vi "Estimate State-Space Model from FRFs.vi"() -> ()   [LabVIEW 2022 SP3]
doc: "This example demonstrates how to use frequency-domain data to estimate a state-space model. \n\n<B>Instructions:</B>\n1) Run this VI.\n2) Observe how the simulated frequency response matches the measured frequency response.\n3) Change the orders of the models, and observe how these changes affect the estimation error."
uses:
  <vilib>/addons/System Identification/Frequency Domain Estimation.llb/SI Estimate Discrete State-Space Model from FRF (SISO Arbitrary).vi
  <vilib>/addons/System Identification/NI_SysID.lvlib
panel:
  in  "name or relative path":path=path "C:/Users/LAV-UFSC/OneDrive - UFSC/Documents/LAV - TCC/Dados-Experimentos/25-04/frf_2.txt"
  in  "noise subspace (%)":dbl=77.0
  in  "FRF format":T1
  out "Phase Response":cluster{"frequency":dbl[], "amplitude":dbl[]}[](graph)
  out "Magnitude Response":cluster{"frequency":dbl[], "amplitude":dbl[]}[](graph)
  in  "Order":i32=67
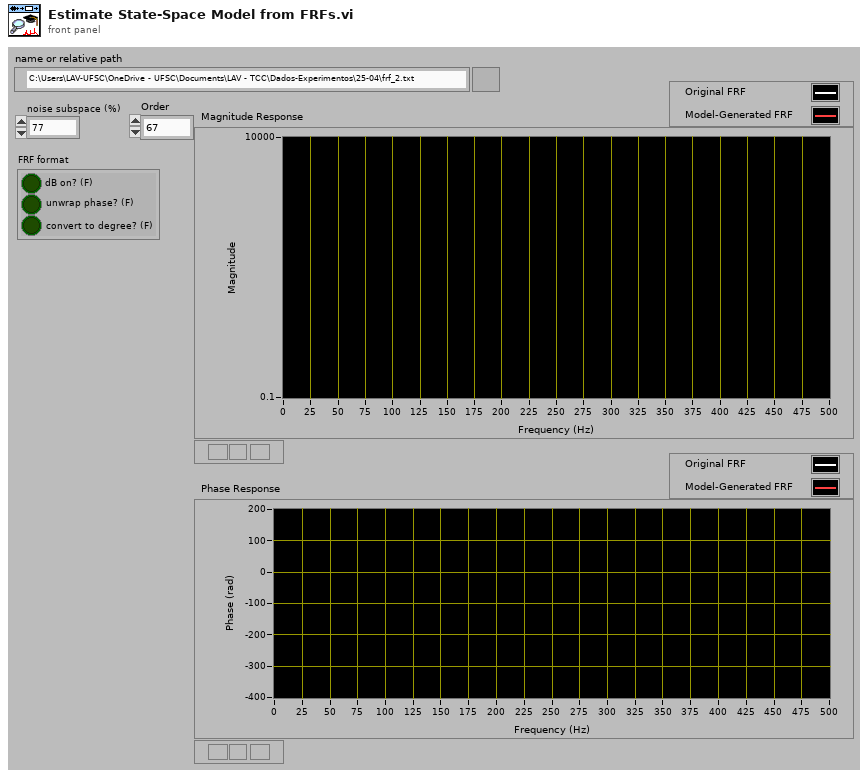
[diagram p1: front panel]
types:
  T1 = cluster{"dB on? (F)":bool, "unwrap phase? (F)":bool, "convert to degree? (F)":bool}
  T2 = cluster{"start frequency":dbl, "end frequency":dbl, "num of freq bins":i32, "interval type":u16}
  T3 = typedef "NI_SysID.lvlib/si_generic model.ctl" = cluster{"attributes":cluster{"version":string, "model type":T4, "input names":string[], "output names":string[], "notes":string}, "coefficients":cluster{"A ":dbl[][][], "B":dbl[][][], "F":dbl[][][], "C":dbl[][][], "D":dbl[][][]}, "std deviations":cluster{"A ":dbl[][][], "B":dbl[][][], "F":dbl[][][], "C":dbl[][][], "D":dbl[][][]}, "coefficients covariance":dbl[][][], "noise variance":dbl[][], "fs":dbl, "system info":cluster{"number of inputs":i32, "number of outputs":i32, "A order":i32[][], "B order":i32[][], "F order":i32[][], "C order":i32[][], "D order":i32[][], "Delays":i32[][]}, "kalman gain":dbl[][], "initial state":dbl[], "trans func":cluster{"betas":dbl[], "alphas":dbl[]}[][], "zeros-poles":cluster{"zeros":cdb[], "poles":cdb[], "gain":dbl}[][], "std of trans func":cluster{"betas":dbl[], "alphas":dbl[]}[][], "std of zeros-poles":cluster{"zeros":cdb[], "poles":cdb[], "gain":dbl}[][], "trans func (noise)":cluster{"betas":dbl[], "alphas":dbl[]}[][], "std of trans func (noise)":cluster{"betas":dbl[], "alphas":dbl[]}[][], "zeros-poles (noise)":cluster{"zeros":cdb[], "poles":cdb[], "gain":dbl}[][], "std of zeros-poles (noise)":cluster{"zeros":cdb[], "poles":cdb[], "gain":dbl}[][], "Symbolic State Space Model":cluster{"Symbolic A":string[][], "Symbolic B":string[][], "Symbolic C":string[][], "Symbolic D":string[][], "Symbolic K":string[][], "Symbolic Initial State":string[]}, "delay":dbl[][], "variables":T5, "grey trans func spec":cluster{"orders of TF model":cluster{" num order":i32, "den order":i32}, "# of zeros/poles at origin":cluster{"zeros/poles":u16, "number ":i32}, "delay initial?":bool, "gain initial?":bool}}
  T4 = typedef "NI_SysID.lvlib/SI Model Type.ctl" = u16
  T5 = typedef "NI_SysID.lvlib/si_variables.ctl" = cluster{"name":string, "initial guess":dbl, "upper limit":dbl, "lower limit":dbl, "value":dbl}[]
  T6 = typedef "NI_SysID.lvlib/si_Bode Phase Plot.ctl" = cluster{"frequency":dbl[], "amplitude":dbl[]}[]
  T7 = typedef "NI_SysID.lvlib/si_Bode Magnitude Plot.ctl" = cluster{"frequency":dbl[], "amplitude":dbl[]}[]
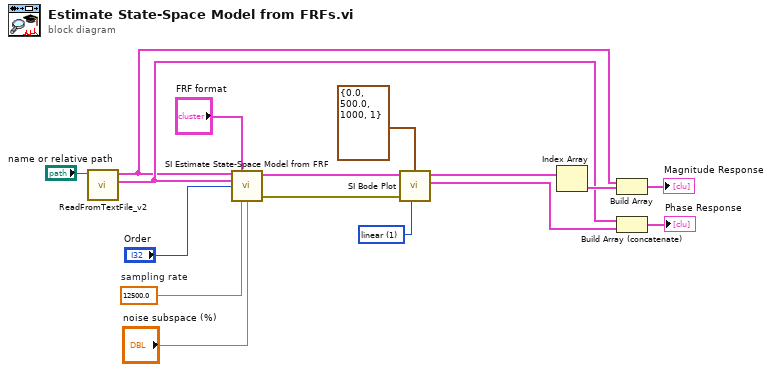
[diagram p0: block diagram]
diagram:
  w12 = 12500.0  # sampling rate
  w3 = u16 1 items=["dB", "linear"] ("magnitude unit")
  n1 = call "ReadFromTextFile_v2.vi"("name or relative path"="name or relative path") -> ("Phase"=w6:cluster{dbl[], dbl[]}, "Magnitude"=w2:cluster{dbl[], dbl[]})  [unwired: 6 in, 2 out]
  n2 = call-poly <vilib>:"SI Estimate State-Space Model from FRF.vi"("FRF magnitude"=w2, "FRF format"="FRF format", "FRF phase"=w6, "number of states"="Order", "sampling rate (Hz)"=w12, "noise subspace (%)"="noise subspace (%)") -> ("system model out"=w15:T3, "error out"=w4:errorcluster)  [unwired: 2 in, 6 out]
  n3 = call <vilib>:"SI Bode Plot.vi"("magnitude unit"=w3, "freq info"=T2 {"start frequency"=0.0, "end frequency"=500.0, "num of freq bins"=1000, "interval type"=1}, "error in (no error)"=w4, "system model"=w15) -> ("Bode phase plot"=w1:T6, "Bode magnitude plot"=w13:T7)  [unwired: 3 in, 3 out]
  n4 = Index Array(array=w13) -> (element=w11:cluster{"frequency":dbl[], "amplitude":dbl[]})  [unwired: 1 in]
  n5 = Build Array(w2, w11) -> (→"Magnitude Response":cluster{"frequency":dbl[], "amplitude":dbl[]}[])
  n6 = Build Array (concatenate)(w6, w1) -> (→"Phase Response":T6)
